vi "Read File.vi"(8 "error in (no error)":errorcluster, 11 "Spreadsheet in":refnum<class "Spreadsheet.lvclass">) -> (0 "error out":errorcluster, 2 "File":path, 3 "Spreadsheet out":refnum<class "Spreadsheet.lvclass">)   [LabVIEW 2013, in "Spreadsheet.lvclass"]
uses:
  Spreadsheet.lvclass
  Spreadsheet.lvclass/Spreadsheet.ctl
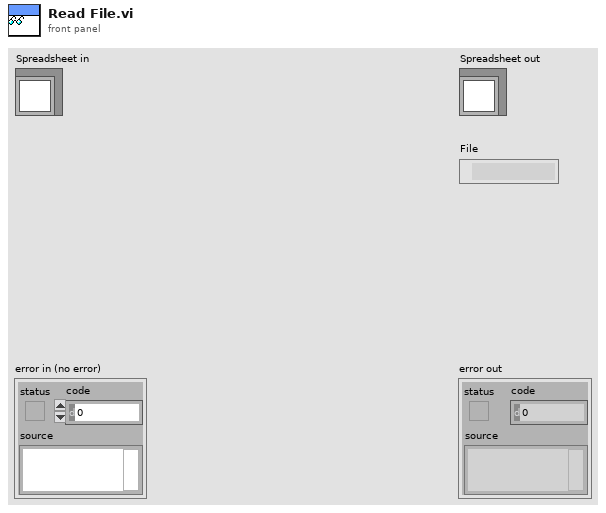
[diagram p1: front panel]
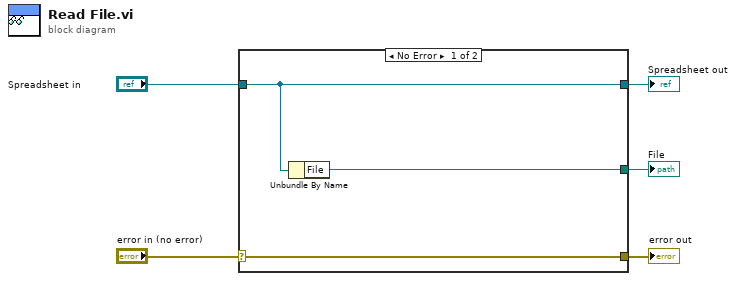
[diagram p0: block diagram]
diagram:
  n1 = case shown="No Error" "error in (no error)" {
    selector: "error in (no error)" -> [w8 w9]
    tunnel: [w8 w9] -> w4
    tunnel: [w7 w10] -> w2
    tunnel: "Spreadsheet in" -> [w7 w10]
    tunnel: [w6 _] -> w1
    frame No Error {
      n2 = Unbundle By Name(w7) -> ("File"=w6:path)
    }
    frame Error {
    }
  }
  "error out" <- w4
  "Spreadsheet out" <- w2
  "File" <- w1
